vi "Add Part to Worksheet.vi"(8 "error in":errorcluster, 10 "PartType":i32(ring) items=["Chart", "Drawings", "ImagePart", "PivotTable", "TableDefinition", "WorksheetComments", "WorksheetDrawing"], 11 "WorksheetPart in":refnum<k24>) -> (0 "error out":errorcluster, 2 "Open Xml Part":refnum<k24>, 3 "WorksheetPart out":refnum<k24>)   [LabVIEW 2019, in "Open Xml.lvlib"]
uses:
  Open Xml.lvlib
  D:/git/Open-Xml-LabVIEW/Source/OpenXmlGenericsWrapper.dll
  OpenXmlGenericsWrapper.dll
  D:/git/Open-Xml-LabVIEW/Source/DocumentFormat.OpenXml.dll
  DocumentFormat.OpenXml.dll
  D:/git/Open-Xml-LabVIEW/Source/DocumentFormat.OpenXml.Framework.dll
  DocumentFormat.OpenXml.Framework.dll
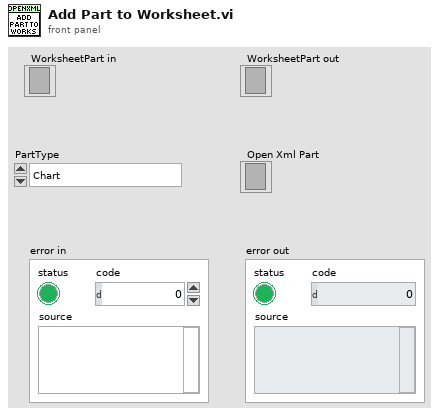
[diagram p1: front panel]
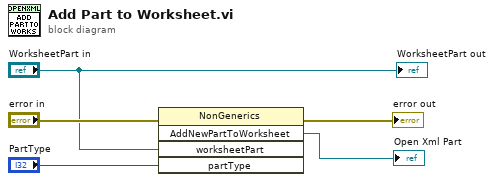
[diagram p0: block diagram]
diagram:
  n1 = invoke class="NonGenerics" method="AddNewPartToWorksheet"(error in="error in", "worksheetPart"="WorksheetPart in", "partType"="PartType") -> (error out=→"error out":errorcluster, "AddNewPartToWorksheet"=→"Open Xml Part":refnum<k24>)  [unwired: 2 in, 3 out]
  "WorksheetPart out" <- "WorksheetPart in"
